vi "手动调试界面.vi"() -> ()   [LabVIEW 2016, in "质控单元.lvlib"]
uses:
  <vilib>/Utility/miscctls.llb/LVPointTypeDef.ctl
panel:
  in  "加标回收流程":bool
  in  "关闭":bool
  in  "总氮停止":bool
  in  "总氮排液":bool
  in  "总氮调试":bool
  in  "CODCr停止":bool
  in  "CODCr排液":bool
  in  "CODCr调试":bool
  in  "CODMn停止":bool
  in  "CODMn排液":bool
  in  "CODMn调试":bool
  in  "总磷停止":bool
  in  "总磷排液":bool
  in  "总磷调试":bool
  in  "氨氮停止":bool
  in  "氨氮排液":bool
  in  "氨氮调试":bool
  # "手动调试界面"
  # "氨氮模块"
  # "总磷模块"
  # "总氮模块"
  # "CODMn模块"
  # "CODCr模块"
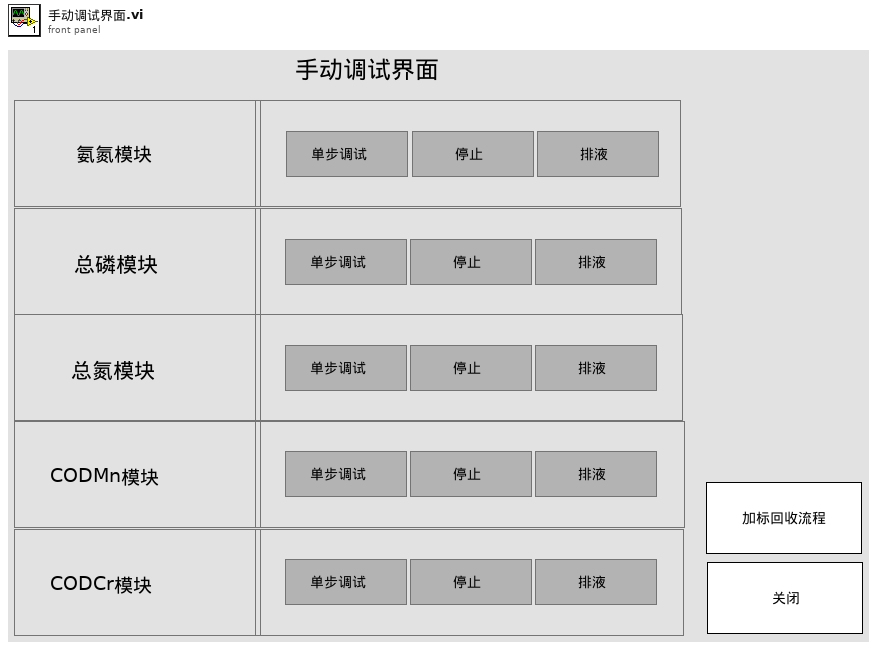
[diagram p1: front panel]
types:
  T1 = typedef "LVPointTypeDef.ctl" = cluster{"Horizontal":i16, "Vertical":i16}
  T2 = cluster{"氨氮":u8, "总磷":u8, "总氮":u8, "CODMn":u8, "CODCr":u8}
  T3 = cluster{"氨氮":bool, "总磷":bool, "总氮":bool, "CODMn":bool, "CODCr":bool}
  T4 = enum32{"Bad", "Idle", "Run top level", "Running"}
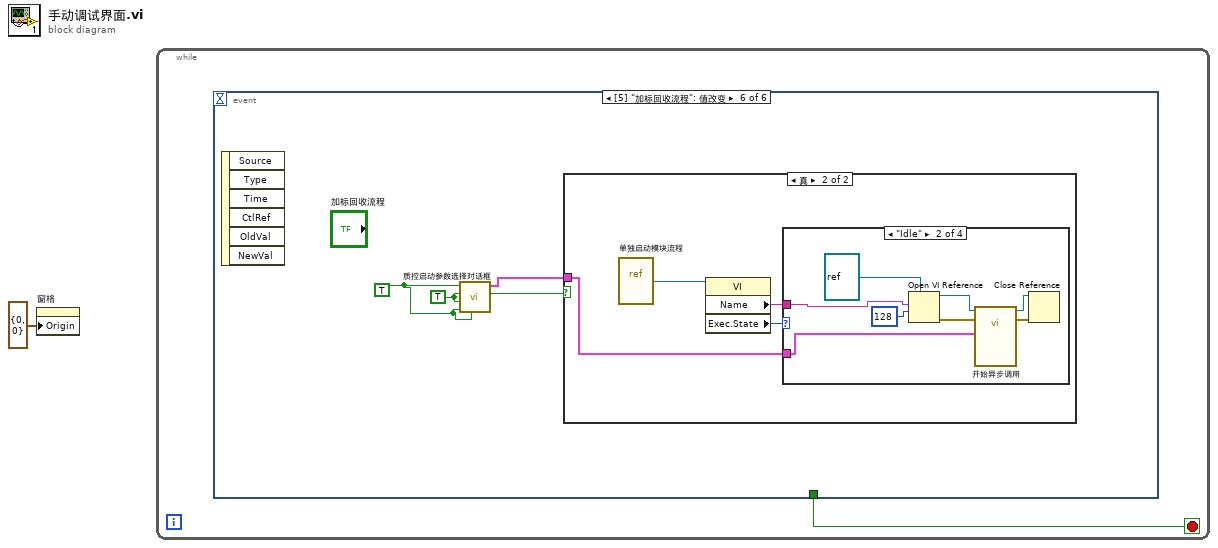
[diagram p0: block diagram]
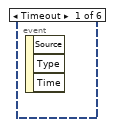
[diagram p2: hidden frame]
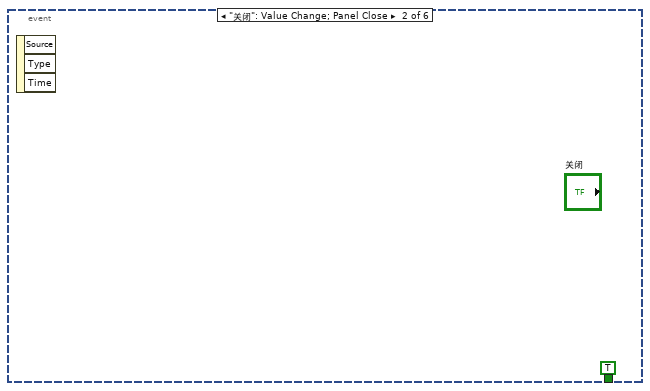
[diagram p3: hidden frame]
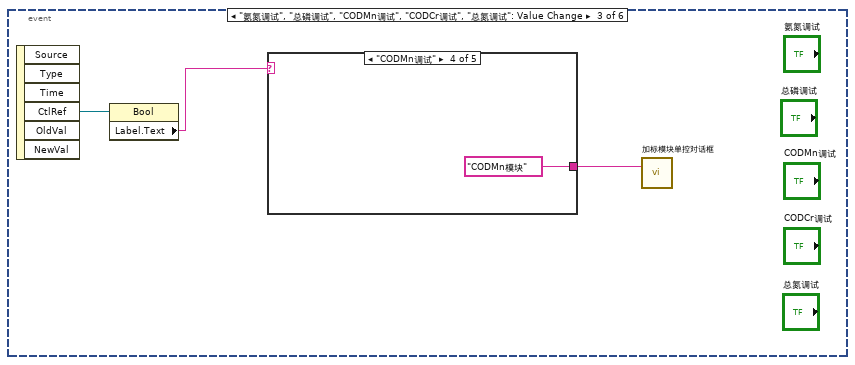
[diagram p4: hidden frame]
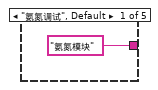
[diagram p5: hidden frame]
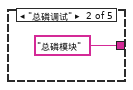
[diagram p6: hidden frame]
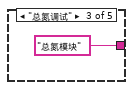
[diagram p7: hidden frame]
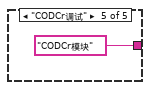
[diagram p8: hidden frame]
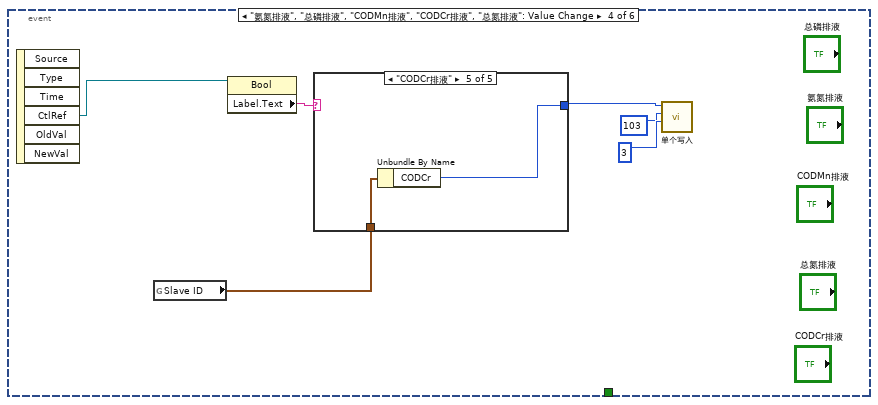
[diagram p9: hidden frame]
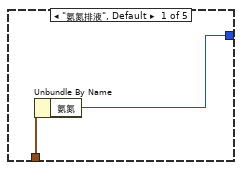
[diagram p10: hidden frame]
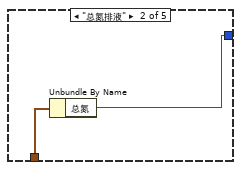
[diagram p11: hidden frame]
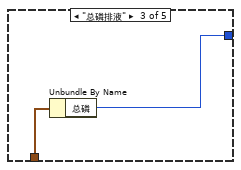
[diagram p12: hidden frame]
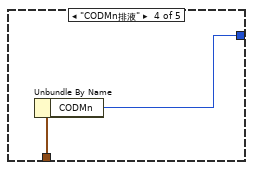
[diagram p13: hidden frame]
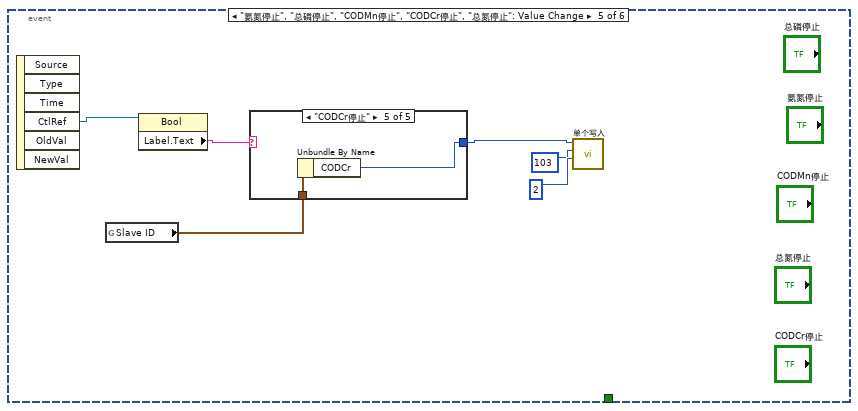
[diagram p14: hidden frame]
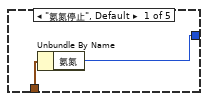
[diagram p15: hidden frame]
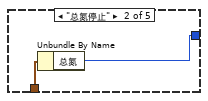
[diagram p16: hidden frame]
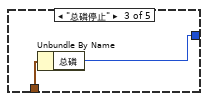
[diagram p17: hidden frame]
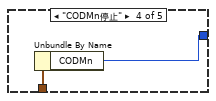
[diagram p18: hidden frame]
diagram:
  n1 = property on="窗格" class="Pane"("Origin"=T1 {"Horizontal"=0, "Vertical"=0} ("原点")) -> ()  [unwired: 2 in, 2 out]
  n2 = while {
    stop <- w2 stop-if-true
    n3 = event shown="[5] \"加标回收流程\": 值改变" {
      selector: _ -> [_ _ _ _ _ _]
      dyn-events: _ -> [_ _ _ _ _ _]
      timeout: _ -> [_ _ _ _ _ _]
      tunnel: [_ TRUE ("关闭") _ _ _ _] -> w2
      event Timeout {
        n4 = event-data() -> ()  [unwired: 1 in, 3 out]
      }
      event "关闭": Value Change; Panel Close {
        n5 = event-data() -> ()  [unwired: 1 in, 3 out]
      }
      event "氨氮调试", "总磷调试", "CODMn调试", "CODCr调试", "总氮调试": Value Change {
        n6 = event-data() -> ("CtlRef"=w5:refnum<vi>)  [unwired: 1 in, 5 out]
        n7 = property class="Bool"(reference=w5) -> ("Label.Text"=w4:string)  [unwired: 1 in, 2 out]
        n8 = case shown="\"CODMn调试\"" w4 {
          tunnel: ["氨氮模块" ("标题") "总磷模块" ("标题") "总氮模块" ("标题") "CODMn模块" ("标题") "CODCr模块" ("标题")] -> w6
          frame "氨氮调试", Default {
          }
          frame "总磷调试" {
          }
          frame "总氮调试" {
          }
          frame "CODMn调试" {
          }
          frame "CODCr调试" {
          }
        }
        n9 = call "加标模块单控对话框.vi"("标题"=w6) -> ()  [unwired: 11 in]
      }
      event "氨氮排液", "总磷排液", "CODMn排液", "CODCr排液", "总氮排液": Value Change {
        n10 = event-data() -> ("CtlRef"=w13:refnum<vi>)  [unwired: 1 in, 5 out]
        n11 = global read "断电保存全局.vi" "Slave ID"() -> (w12:T2)
        n12 = property class="Bool"(reference=w13) -> ("Label.Text"=w17:string)  [unwired: 1 in, 2 out]
        n13 = case shown="\"CODCr排液\"" w17 {
          tunnel: [w18 w20 w22 w24 w26] -> w14
          tunnel: w12 -> [w19 w21 w23 w25 w27]
          frame "氨氮排液", Default {
            n14 = Unbundle By Name(w19) -> ("氨氮"=w18:u8)
          }
          frame "总氮排液" {
            n15 = Unbundle By Name(w21) -> ("总氮"=w20:u8)
          }
          frame "总磷排液" {
            n16 = Unbundle By Name(w23) -> ("总磷"=w22:u8)
          }
          frame "CODMn排液" {
            n17 = Unbundle By Name(w25) -> ("CODMn"=w24:u8)
          }
          frame "CODCr排液" {
            n18 = Unbundle By Name(w27) -> ("CODCr"=w26:u8)
          }
        }
        n19 = call "单个写入.vi"("value"=u16 3, "address"=u16 103, "Slave ID"=w14) -> ()  [unwired: 8 in, 1 out]
      }
      event "氨氮停止", "总磷停止", "CODMn停止", "CODCr停止", "总氮停止": Value Change {
        n20 = event-data() -> ("CtlRef"=w29:refnum<vi>)  [unwired: 1 in, 5 out]
        n21 = global read "断电保存全局.vi" "Slave ID"() -> (w28:T2)
        n22 = property class="Bool"(reference=w29) -> ("Label.Text"=w33:string)  [unwired: 1 in, 2 out]
        n23 = case shown="\"CODCr停止\"" w33 {
          tunnel: [w34 w36 w38 w40 w42] -> w30
          tunnel: w28 -> [w35 w37 w39 w41 w43]
          frame "氨氮停止", Default {
            n24 = Unbundle By Name(w35) -> ("氨氮"=w34:u8)
          }
          frame "总氮停止" {
            n25 = Unbundle By Name(w37) -> ("总氮"=w36:u8)
          }
          frame "总磷停止" {
            n26 = Unbundle By Name(w39) -> ("总磷"=w38:u8)
          }
          frame "CODMn停止" {
            n27 = Unbundle By Name(w41) -> ("CODMn"=w40:u8)
          }
          frame "CODCr停止" {
            n28 = Unbundle By Name(w43) -> ("CODCr"=w42:u8)
          }
        }
        n29 = call "单个写入.vi"("value"=u16 2, "address"=u16 103, "Slave ID"=w30) -> ()  [unwired: 8 in, 1 out]
      }
      event "加标回收流程": Value Change {
        w47 = TRUE ("总氮")
        w46 = TRUE ("氨氮")
        n30 = event-data() -> ()  [unwired: 1 in, 6 out]
        n31 = call "质控启动参数选择对话框.vi"("CODCr"=w46, "CODMn"=w46, "总氮"=w47, "总磷"=w47, "氨氮"=w46) -> ("确定启动"=w45:bool, "启动模块"=w44:T3)  [unwired: 4 in, 1 out]
        n32 = case shown="真" w45 {
          tunnel: w44 -> [_ w48]
          frame False {
          }
          frame True {
            n33 = vi-ref "单独启动模块流程.vi"() -> (w49:refnum<vi>)
            n34 = property class="VI"(reference=w49) -> ("Name"=w51:string, "Exec.State"=w50:T4)  [unwired: 1 in, 2 out]
            n35 = case shown="\"Idle\"" w50 {
              tunnel: w51 -> [_ w55 _ _]
              tunnel: w48 -> [_ w52 _ _]
              frame "Bad", Default {
              }
              frame "Idle" {
                n36 = Open VI Reference(type specifier VI Refnum (for type only)=refnum<vi> refnum ("类型说明符VI引用句柄（仅用于类型）"), vi path=w55, options=128 ("选项")) -> (vi reference=w59:refnum<vi>, error out=w54:errorcluster)  [unwired: 3 in]
                n37 = call-by-ref "开始异步调用"(reference=w59, error in=w54, "模块选择"=w52) -> (reference out=w58:refnum<vi>, error out=w53:errorcluster)  [unwired: 11 in]
                n38 = Close Reference(reference=w58, error in (no error)=w53) -> ()  [unwired: 1 out]
              }
              frame "Run top level" {
              }
              frame "Running" {
              }
            }
          }
        }
      }
    }
  }
